vi "ADO Recordset EOF.vi"(8 "error in (no error)":errorcluster, 11 "ADODB._Recordset In":refnum<k7>) -> (0 "error out":errorcluster, 2 "EOF":bool, 3 "ADODB._Recordset Out":refnum<k7>)   [LabVIEW 2013]
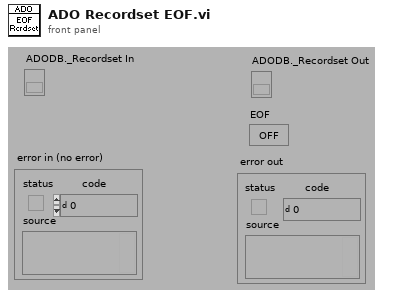
[diagram p1: front panel]
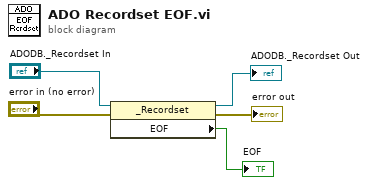
[diagram p0: block diagram]
diagram:
  n1 = property class="_Recordset"(reference="ADODB._Recordset In", error in="error in (no error)") -> (reference out=→"ADODB._Recordset Out":refnum<k7>, error out=→"error out":errorcluster, "EOF"=→"EOF":bool)
